vi "Add.vi"(10 "y":dbl, 11 "x":dbl) -> (3 "x+y":dbl)   [LabVIEW 2015]
doc: "Use the LabVIEW Unit Test Framework Toolkit to check this VI for functional correctness. The test file for this VI, Add.lvtest, is configured to pass."
panel:
  # "Overview: Use the LabVIEW Unit Test Framework Toolkit to check this VI for functional correctness. \nRequirements: LabVIEW Full Development System, Unit Test Framework Toolkit\nInstructions:\n1.  Execute the Add.lvtest test file for this VI. In the Project Explorer window, expand the Unit Test Files folder, right-click Add.lvtest, and select Run from the shortcut menu.\n2.  View the test results in the Unit Test Frameworks Results window, which shows that this test passes."
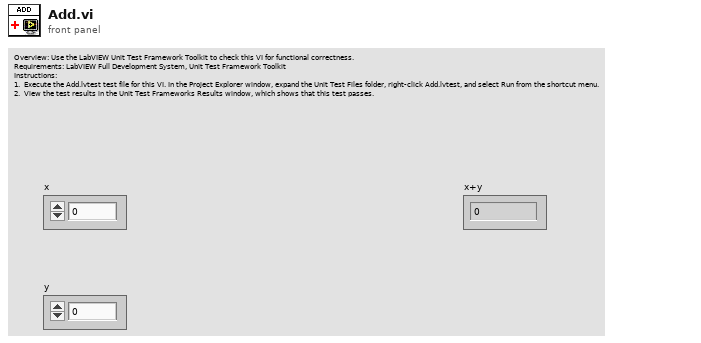
[diagram p1: front panel]
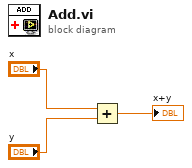
[diagram p0: block diagram]
diagram:
  n1 = Add(x="x", y="y") -> (x+y=→"x+y":dbl)
